vi "Sorted ID With Task Name.vi"(8 "error in (no error)":errorcluster, 11 "Composite Map Task in":refnum<class "Composite ID-Map Task.lvclass">) -> (0 "error out":errorcluster, 2 "Items":string[](array[string]), 3 "Composite Map Task out":refnum<class "Composite ID-Map Task.lvclass">)   [LabVIEW 2024, in "Composite ID-Map Task.lvclass"]
uses:
  Composite ID-Map Task.lvclass
  Composite ID-Map Task.lvclass/Composite ID-Map Task.ctl
  Task Ancestor/Task Ancestor.lvclass/Task Ancestor.ctl
  196ac749-0515-4661-a884-ad860d762ac1.vi
  Task Ancestor/Public Data/Read Task Name.vi
  <vilib>/Comparison/Less/Less Functor/Less Functor.lvclass
  Task Ancestor/Task Ancestor.lvclass
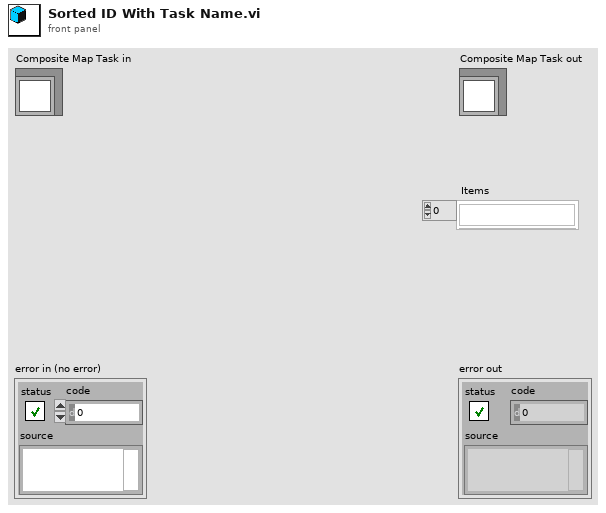
[diagram p1: front panel]
types:
  T1 = cluster{"ID":i64, "Task":refnum<class "Task Ancestor.lvclass">}
  T2 = cluster{"ID":i64, "Task":refnum<class "Task Ancestor.lvclass">}[]
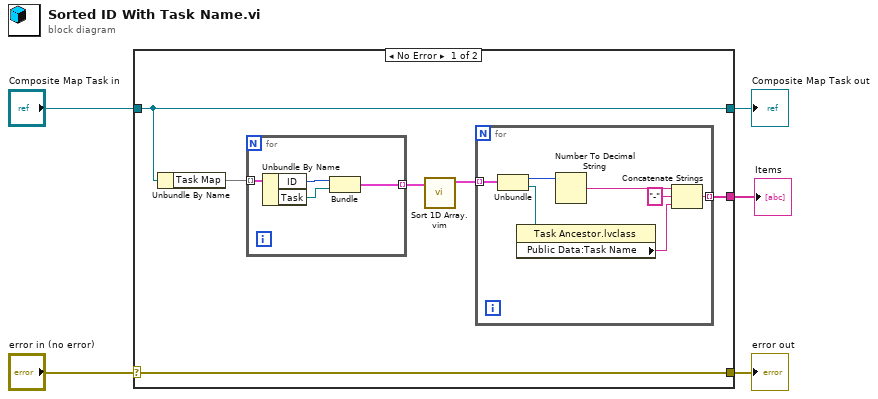
[diagram p0: block diagram]
diagram:
  n1 = case shown="No Error" "error in (no error)" {
    selector: "error in (no error)" -> [w11 w24]
    tunnel: [w11 w24] -> w4
    tunnel: [w10 w23] -> w2
    tunnel: "Composite Map Task in" -> [w10 w23]
    tunnel: [w6 _] -> w1
    frame No Error {
      n2 = Unbundle By Name(w10) -> ("Task Map"=w9:map{i64, refnum<class "Task Ancestor.lvclass">})
      n3 = for {
        tunnel: w9 -> [w22] mode=indexing
        tunnel: [w19] -> w8 mode=indexing
        n4 = Unbundle By Name(w22) -> ("ID"=w21:i64, "Task"=w20:refnum<class "Task Ancestor.lvclass">)
        n5 = Bundle("ID"=w21, "Task"=w20) -> (w19:T1)  [unwired: 1 in]
      }
      n6 = call "Sort 1D Array.vim"("unsorted array"=w8) -> ("sorted array"=w7:T2)  [unwired: 10 in]
      n7 = for {
        tunnel: w7 -> [w18] mode=indexing
        tunnel: [w12] -> w6 mode=indexing
        n8 = Unbundle(w18) -> ("ID"=w17:i64, "Task"=w15:refnum<class "Task Ancestor.lvclass">)
        n9 = property class="Task Ancestor.lvclass"(reference=w15) -> ("Public Data:Task Name"=w13:string)  [unwired: 1 in, 2 out]
        n10 = Number To Decimal String(number=w17) -> (decimal integer string=w16:string)  [unwired: 1 in]
        n11 = Concatenate Strings(w16, "-" ("string"), w13) -> (w12:string)
      }
    }
    frame Error {
    }
  }
  "error out" <- w4
  "Composite Map Task out" <- w2
  "Items" <- w1
